vi "Detect Circles.vi"() -> ()   [LabVIEW 2020, in "examples.lvlib"]
uses:
  examples.lvlib
  feature_detection/Hough Circle Result.ctl
  common/Image Point (Float).ctl
  image/Kernel Block Size.ctl
  feature_detection/Hough Circle Parameters.ctl
  feature_detection/Hough Circle Modes.ctl
  image/Canny Aperture Size.ctl
  image/ARGB Colour.ctl
  image/New Image (ARGB Preallocated).vi
  image/Copy Pixmap to Image (ARGB Flatten Mask).vi
  image/Draw Image to Picture (ARGB).vi
  image/Blur (Gaussian Greyscale).vi
  image/Threshold (Binary).vi
  image/Draw Image to Picture (Greyscale).vi
  image/Draw Circle (ARGB).vi
  image/New Image (ARGB Preallocated).vi/3321fa97-f432-4e1e-8db9-a0df79aed21b.vi
  image/ARGB Colour to U32 Pixel Value.vi
  image/Copy Pixmap to Image (ARGB Flatten Mask).vi/7d03ccf7-b889-4e8d-9f2a-57831e73dbde.vi
  image/Draw Image to Picture (ARGB).vi/8cd07b1b-062e-4fe4-9e87-2eb3dc89fe0e.vi
  image/New Image (Greyscale Preallocated).vi/6598b9e0-8a08-46f5-91fd-ca1b87217137.vi
  image/ARGBExtractChannel.vi
  image/Blur (Gaussian Greyscale).vi/68bb216c-d3e3-4366-946f-f5b7f5c74ae7.vi
  image/ThresholdCore.vi
  image/Draw Image to Picture (Greyscale).vi/9ae995ca-ccda-485c-89ac-02736fde3e8e.vi
  image/Draw Circle (ARGB).vi/8336a1cf-e433-4bea-8080-376bdb783d4e.vi
  image/FixPixmap.vi
  image/Default8bitColourMap.vi
  <vilib>/Utility/error.llb/Error Cluster From Error Code.vi
  image/image.lvlib
  feature_detection/feature_detection.lvlib
  common/common.lvlib
panel:
  in  "Image to Binary Mode":enum16{"Threshold", "Canny Edges"}(ring)=enum."Canny Edges"
  out "Results":T1[](array[typedef])
  out "Input":picture
  out "Blur & Binary":picture
  out "Draw Overlay":picture
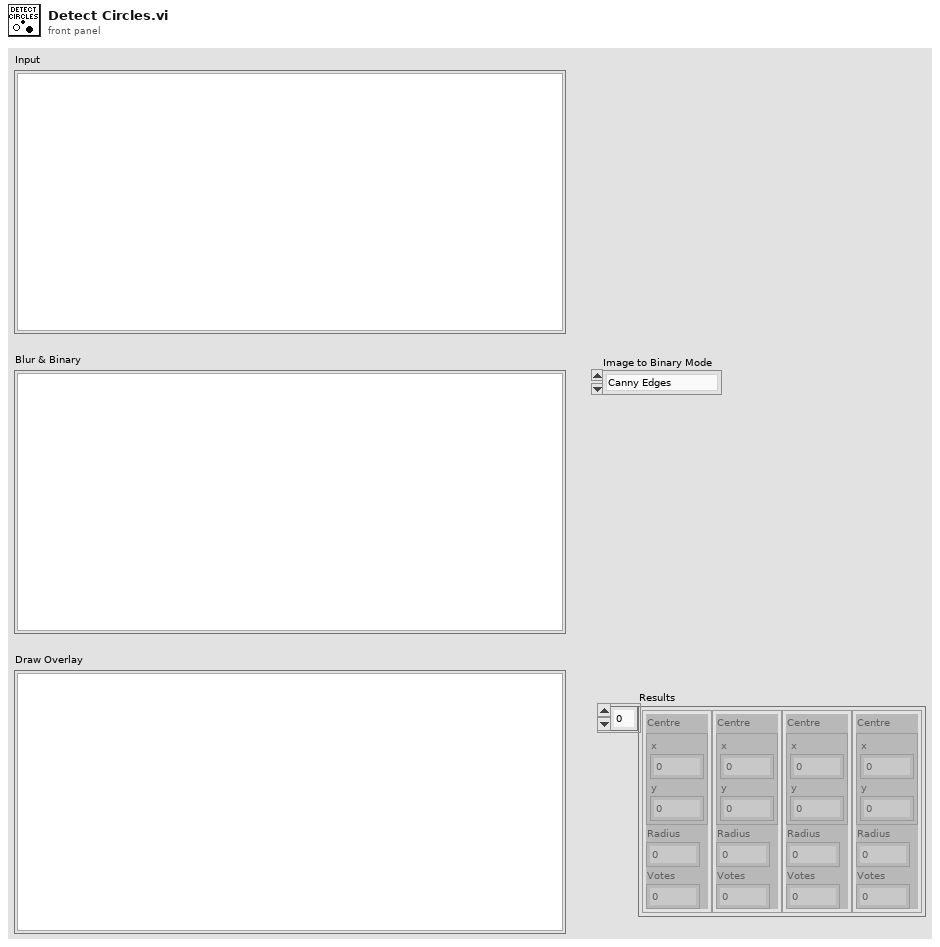
[diagram p1: front panel]
types:
  T1 = typedef "feature_detection.lvlib/Hough Circle Result.ctl" = cluster{"Centre":T2, "Radius":dbl, "Votes":dbl}
  T2 = typedef "common.lvlib/Image Point (Float).ctl" = cluster{"x":dbl, "y":dbl}
  T3 = typedef "feature_detection.lvlib/Hough Circle Modes.ctl" = enum16{"GRADIENT", "GRADIENT_ALT"}
  T4 = typedef "feature_detection.lvlib/Hough Circle Parameters.ctl" = cluster{"Param1":dbl, "Param2":dbl, "Minimum Radius":i32, "Maximum Radius":i32}
  T5 = typedef "image.lvlib/Kernel Block Size.ctl" = enum16{"3", "5", "7", "9", "11", "13", "15", "17", "19", "21", "23", "25", "27", "29", "31", "33", "35", "37", "39", "41", "43", "45", "47", "49", "51", "53", "55", "57", "59", "61", "63", "65", "67", "69", "71", "73", "75", "77", "79", "81", "83", "85", "87", "89", "91", "93", "95", "97", "99", "101", "103", "105", "107", "109", "111", "113", "115", "117", "119", "121", "123", "125", "127", "129", "131", "133", "135", "137", "139", "141", "143", "145", "147", "149", "151", "153", "155", "157", "159", "161", "163", "165", "167", "169", "171", "173", "175", "177", "179", "181", "183", "185", "187", "189", "191", "193", "195", "197", "199", "201", "203", "205", "207", "209", "211", "213", "215", "217", "219", "221", "223", "225", "227", "229", "231", "233", "235", "237", "239", "241", "243", "245", "247", "249", "251", "253", "255", "257", "259", "261", "263", "265", "267", "269", "271", "273", "275", "277", "279", "281", "283", "285", "287", "289", "291", "293", "295", "297", "299", "301", "303", "305", "307", "309", "311", "313", "315", "317", "319", "321", "323", "325", "327", "329", "331", "333", "335", "337", "339", "341", "343", "345", "347", "349", "351", "353", "355", "357"}
  T6 = typedef "imagedata.ctl" = cluster{"image type":i32, "image depth":i32, "image":u8[], "mask":u8[], "colors":u32[], "Rectangle":cluster{"left":i16, "top":i16, "right":i16, "bottom":i16}}
  T7 = typedef "image.lvlib/ARGB Image.ctl" = refnum<data-value>
  T8 = typedef "image.lvlib/Greyscale Image.ctl" = refnum<data-value>
  T9 = typedef "image.lvlib/Canny Aperture Size.ctl" = enum16{"3", "5", "7"}
  T10 = typedef "image.lvlib/ARGB Colour.ctl" = cluster{"Alpha":u8, "RGB":u32}
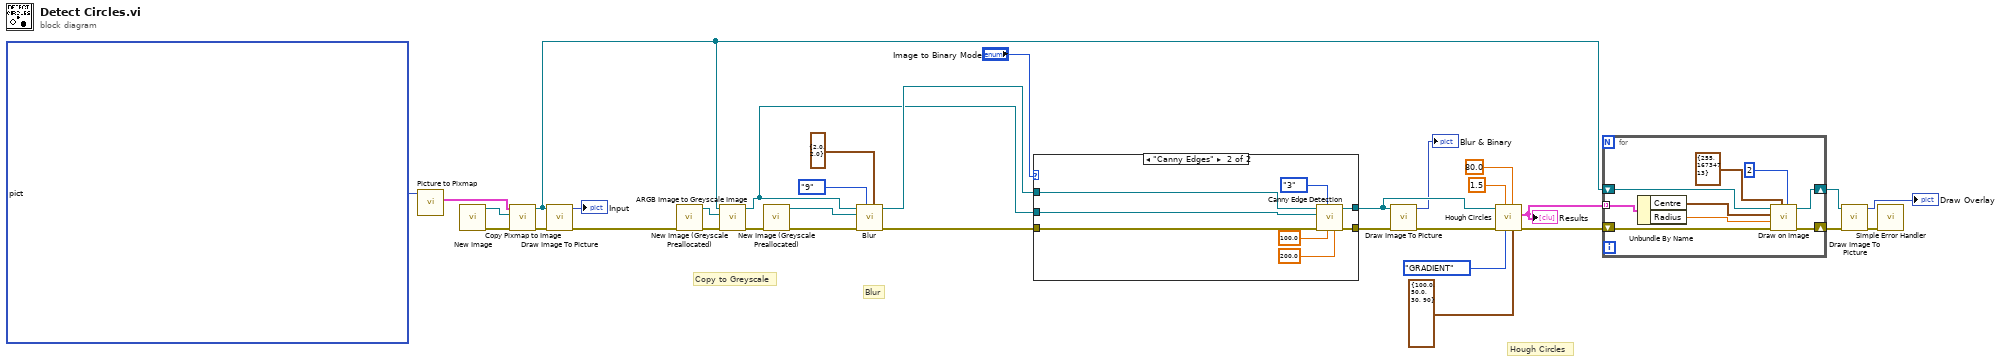
[diagram p0: block diagram]
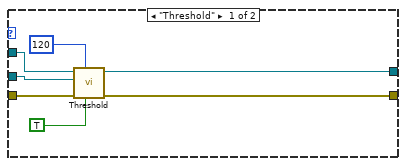
[diagram p2: hidden frame]
diagram:
  # "Hough Circles"
  # "Blur"
  # "Copy to Greyscale"
  n1 = call <vilib>:"Picture to Pixmap.vi"("picture"=picture bytes[518430] ("Input")) -> ("image data"=w1:T6)  [unwired: 9 in, 1 out]
  n2 = call-poly "New Image.vi"() -> ("error out"=w32:errorcluster, "ARGB Image"=w33:T7)  [unwired: 10 in]
  n3 = call-poly "Copy Pixmap to Image.vi"("error in (no error)"=w32, "ARGB Image Destination in"=w33, "Pixmap Image Data"=w1) -> ("error out"=w22:errorcluster, "ARGB Image Destination"=w23:T7)  [unwired: 7 in]
  n4 = call-poly "Draw Image To Picture.vi"("error in (no error)"=w22, "ARGB Image Source in"=w23) -> ("error out"=w21:errorcluster, "Picture"=→"Input":picture)  [unwired: 8 in]
  n5 = call "New Image (Greyscale Preallocated).vi"("error in (no error)"=w21) -> ("error out"=w27:errorcluster, "Greyscale Image"=w26:T8)  [unwired: 9 in]
  n6 = call "ARGB Image to Greyscale Image.vi"("error in (no error)"=w27, "Greyscale Image Destination in"=w26, "ARGB Image Source in"=w23) -> ("error out"=w15:errorcluster, "Greyscale Image Destination"=w4:T8)  [unwired: 7 in]
  n7 = call "New Image (Greyscale Preallocated).vi"("error in (no error)"=w15) -> ("error out"=w14:errorcluster, "Greyscale Image"=w12:T8)  [unwired: 9 in]
  n8 = call-poly "Blur.vi"("Sigma"=T2 {"x"=2.0, "y"=2.0}, "Kernel Block Size"=Kernel_Block_Size."9", "error in (no error)"=w14, "Gaussian Blur Result in"=w12, "Greyscale Image-Source in"=w4) -> ("error out"=w5:errorcluster, "Gaussian Blur Result"=w13:T8)  [unwired: 5 in]
  n9 = case shown="\"Canny Edges\"" "Image to Binary Mode" {
    tunnel: [w35 w48] -> w20
    tunnel: [w36 w47] -> w18
    tunnel: w13 -> [w38 w46]
    tunnel: w5 -> [w39 w45]
    tunnel: w4 -> [w37 w44]
    frame "Threshold" {
      n10 = call-poly "Threshold.vi"("Invert? (Default: False)"=TRUE, "Threshold"=u8 120, "error in (no error)"=w39, "Threshold Result in"=w37, "Greyscale Image-Source in"=w38) -> ("error out"=w35:errorcluster, "Threshold Result"=w36:T8)  [unwired: 5 in]
    }
    frame "Canny Edges" {
      n11 = call "Canny Edge Detection.vi"("Threshold 2"=200.0, "Threshold 1"=100.0, "Aperture Size"=Canny_Aperture_Size."3", "error in (no error)"=w45, "Canny Edge Result in"=w44, "Greyscale Image-Source in"=w46) -> ("error out"=w48:errorcluster, "Canny Edge"=w47:T8)  [unwired: 4 in]
    }
  }
  n12 = call-poly "Draw Image To Picture.vi"("error in (no error)"=w20, "Greyscale Image Source in"=w18) -> ("error out"=w19:errorcluster, "Picture"=→"Blur & Binary":picture)  [unwired: 8 in]
  n13 = call "Hough Circles.vi"("Hough Circle Parameters (Default: OpenCV Defaults)"=T4 {"Param1"=100.0, "Param2"=50.0, "Minimum Radius"=30, "Maximum Radius"=90}, "Minimum Distance"=80.0, "Hough Circle Modes (Default: GRADIENT)"=Hough_Circle_Modes."GRADIENT", "DP"=1.5, "error in (no error)"=w19, "Greyscale Image in"=w18) -> ("error out"=w29:errorcluster, "Results"=w28:T1[])  [unwired: 3 in, 1 out]
  "Results" <- w28
  n14 = for {
    shift-right: [w57] -> w30
    shift-left: w29 -> [w51]
    tunnel: w28 -> [w56] mode=indexing
    shift-right: [w55] -> w25
    shift-left: w23 -> [w52]
    n15 = Unbundle By Name(w56) -> ("Centre"=w54:T2, "Radius"=w53:dbl)
    n16 = call-poly "Draw on Image.vi"("Thickness (Default: 1)"=2, "ARGB Colour"=T10 {"Alpha"=255, "RGB"=16734713}, "error in (no error)"=w51, "Radius"=w53, "Centre"=w54, "ARGB Image in"=w52) -> ("error out"=w57:errorcluster, "ARGB Image"=w55:T7)  [unwired: 4 in]
  }
  n17 = call-poly "Draw Image To Picture.vi"("error in (no error)"=w30, "ARGB Image Source in"=w25) -> ("error out"=w24:errorcluster, "Picture"=→"Draw Overlay":picture)  [unwired: 8 in]
  n18 = call <vilib>:"Simple Error Handler.vi"("error in (no error)"=w24) -> ()  [unwired: 4 in, 5 out]
